vi "2d to 1d.vi"(8 "index":i32, 11 "array":dbl[][](array[numeric])) -> (3 "output array":dbl[](array[numeric]))   [LabVIEW 2013, in "OD600.lvlib" / "OD600.lvclass"]
uses:
  OD600.lvclass
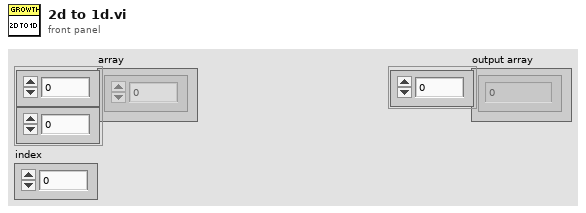
[diagram p1: front panel]
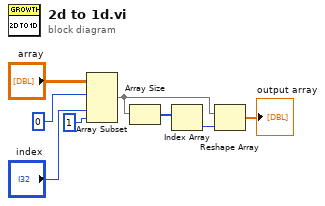
[diagram p0: block diagram]
diagram:
  n1 = Array Subset(array="array", index (row)=0, index (col)="index", length (col)=1) -> (w7:dbl[][])  [unwired: 1 in]
  n2 = Array Size(array=w7) -> (size(s)=w6:i32[])
  n3 = Index Array(array=w6) -> (element=w5:i32)  [unwired: 1 in]
  n4 = Reshape Array(w7, w5) -> (→"output array":dbl[])
